vi "CSV_Reader_v1.vi"(8 "error in (no error)":errorcluster, 11 "CSV Reader Inputs":T2={"Frequency Type"=enum."Frequency", "Measurement Type"=enum."Power", "Digital Channel Selector"=enum."2", "Format Type"=enum."Format B", "CSV File Input"=path ""}) -> (0 "error out":errorcluster, 3 "Terminals":T1[](array[typedef]))   [LabVIEW 2017]
uses:
  CSV Reader Inputs.ctl
  Frequency_Type.ctl
  Measurement_Type.ctl
  Digital Channel Selector.ctl
  Terminal Data v1.ctl
  <vilib>/Utility/file.llb/Read Delimited Spreadsheet (string).vi
panel:
  in  "stop":bool
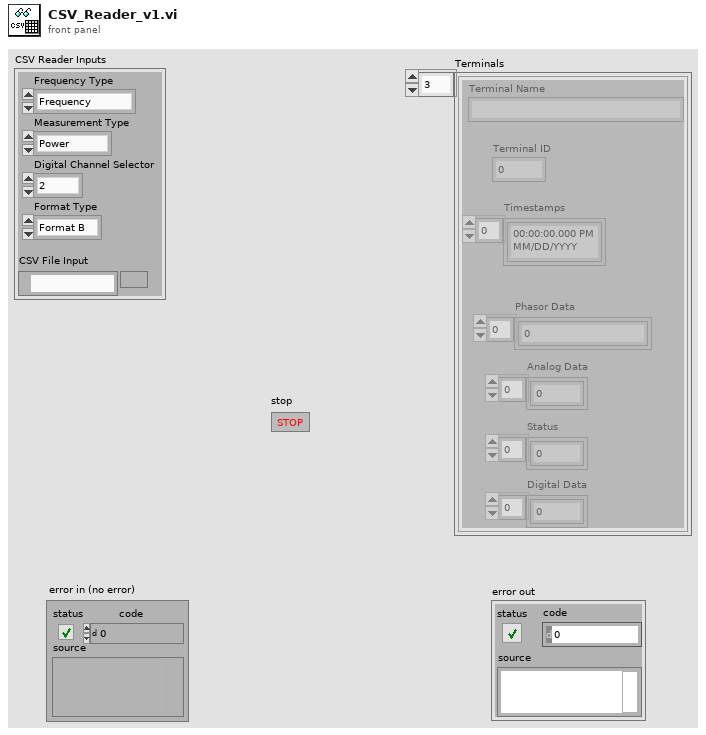
[diagram p1: front panel]
types:
  T1 = typedef "Terminal Data v1.ctl" = cluster{"Terminal Name":string, "Terminal ID":dbl, "Timestamps":timestamp[], "Phasor Data":cdb[], "Analog Data":dbl[], "Status":dbl[], "Digital Data":dbl[]}
  T2 = typedef "CSV Reader Inputs.ctl" = cluster{"Frequency Type":T3, "Measurement Type":T4, "Digital Channel Selector":T5, "Format Type":enum16{"Format A", "Format B"}, "CSV File Input":path}
  T3 = typedef "Frequency_Type.ctl" = enum16{"Frequency", "df/dt"}
  T4 = typedef "Measurement_Type.ctl" = enum16{"Voltage", "Current", "Power"}
  T5 = typedef "Digital Channel Selector.ctl" = enum16{"1", "2", "3"}
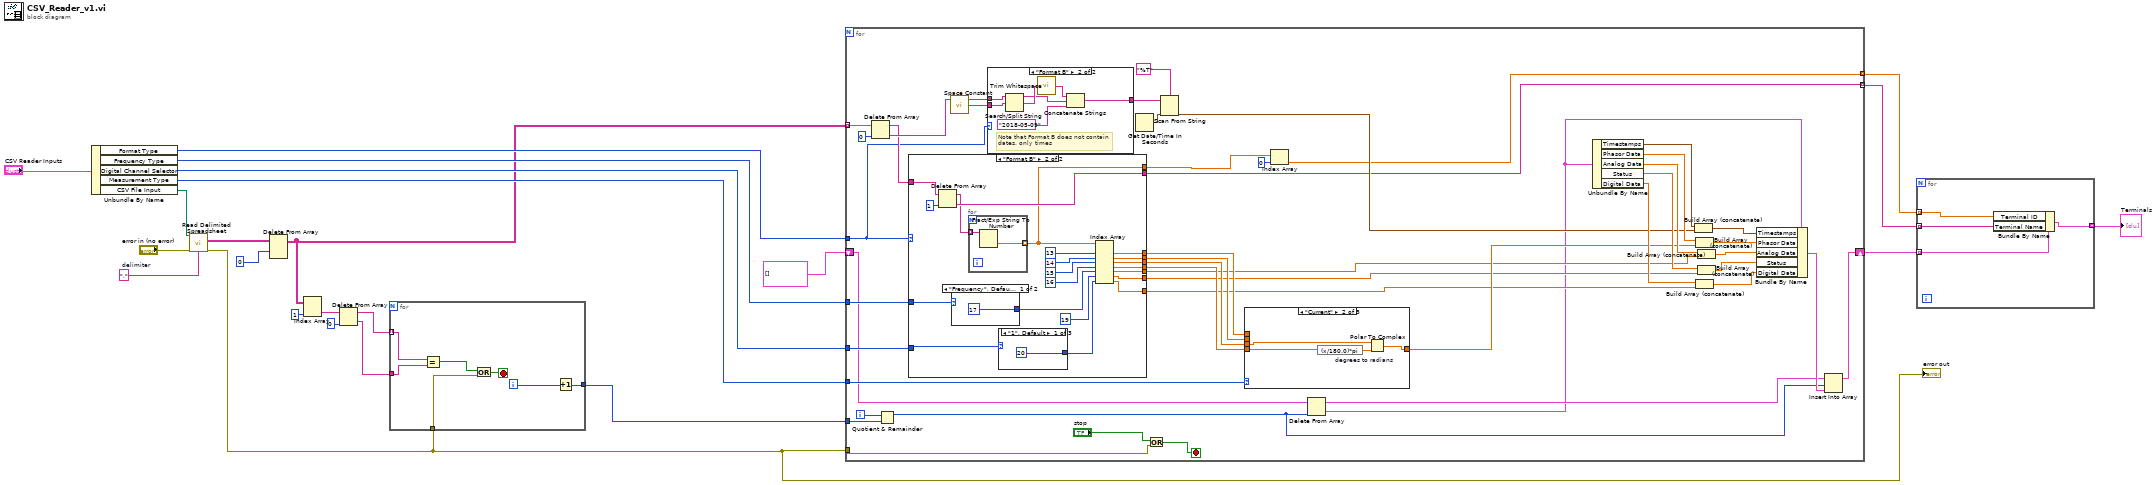
[diagram p0: block diagram]
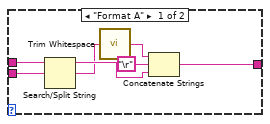
[diagram p2: hidden frame]
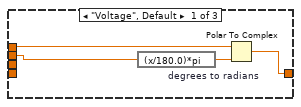
[diagram p3: hidden frame]
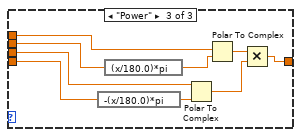
[diagram p4: hidden frame]
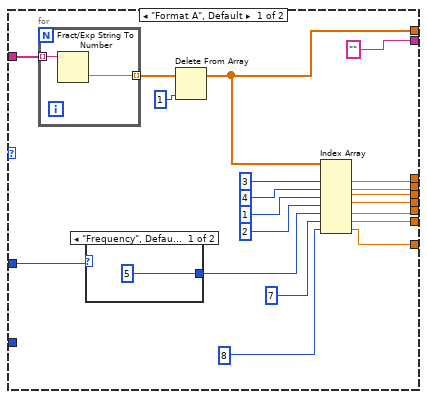
[diagram p5: hidden frame]
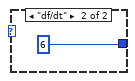
[diagram p6: hidden frame]
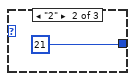
[diagram p7: hidden frame]
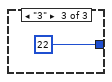
[diagram p8: hidden frame]
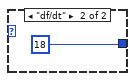
[diagram p9: hidden frame]
diagram:
  w23 = ","  # delimiter
  n1 = Unbundle By Name("CSV Reader Inputs") -> ("Format Type"=w19:enum16{"Format A", "Format B"}, "Frequency Type"=w18:T3, "Digital Channel Selector"=w17:T5, "Measurement Type"=w16:T4, "CSV File Input"=w1:path)
  n2 = call-poly <vilib>:"Read Delimited Spreadsheet.vi"("file path (dialog if empty)"=w1, "error in (no error)"="error in (no error)", "delimiter (\\t)"=w23) -> ("all rows"=w22:string[][], "error out"=w7:errorcluster)  [unwired: 7 in, 4 out]
  "error out" <- w7
  n3 = Delete From Array(array=w22, index (row)=0) -> (array with subset deleted=w14:string[][])  [unwired: 2 in, 1 out]
  n4 = Index Array(array=w14, index (col)=1 ("disabled index (col)")) -> (element=w12:string[])  [unwired: 1 in]
  n5 = Delete From Array(array=w12, index=0) -> (deleted portion=w9:string, array with subset deleted=w10:string[])  [unwired: 1 in]
  n6 = for {
    tunnel: w10 -> [w28] mode=indexing
    tunnel: w9 -> [w27]
    tunnel: [w29] -> w8
    tunnel: w7 -> [w26]
    i -> [w30]
    stop <- w24 stop-if-true
    n7 = Equal?(x=w28, y=w27) -> (x = y?=w25:bool)
    n8 = Or(x=w25, y=w26) -> (x .or. y?=w24:bool)
    n9 = Increment(x=w30) -> (x+1=w29:i32)
  }
  n10 = for {
    tunnel: w14 -> [w72] mode=indexing
    tunnel: w19 -> [w31]
    tunnel: w16 -> [w66]
    tunnel: w18 -> [w61]
    tunnel: w17 -> [w60]
    tunnel: w7 -> [w37]
    shift-right: [w43] -> w5
    shift-left: T1[] [] ("Terminals 2") -> [w41]
    tunnel: w8 -> [w39]
    tunnel: [w33] -> w3 mode=indexing
    tunnel: [w32] -> w4 mode=indexing
    i -> [w45]
    stop <- w36 stop-if-true
    n11 = Delete From Array(array=w72, index=0) -> (deleted portion=w70:string, array with subset deleted=w69:string[])  [unwired: 1 in]
    n12 = Quotient & Remainder(x=w45, y=w39) -> (x-y*floor(x/y)=w40:i32)  [unwired: 1 out]
    n13 = case shown="\"Format B\"" w31 {
      tunnel: w69 -> [w127 w151]
      tunnel: ["" ("String") w150] -> w32
      tunnel: [w108 w148] -> w68
      tunnel: [w118 w143] -> w65
      tunnel: [w117 w142] -> w64
      tunnel: [w116 w141] -> w63
      tunnel: [w115 w140] -> w62
      tunnel: w61 -> [w119 w139]
      tunnel: [w114 w137] -> w51
      tunnel: w60 -> [_ w135]
      tunnel: [w113 w133] -> w49
      tunnel: [w112 w132] -> w47
      frame "Format A", Default {
        n14 = for {
          tunnel: [w130] -> w110 mode=indexing
          tunnel: w127 -> [w131] mode=indexing
          n15 = Fract/Exp String To Number(string=w131) -> (number=w130:dbl)  [unwired: 3 in, 1 out]
        }
        n16 = case shown="\"Frequency\", Default" w119 {
          tunnel: [5 ("index") 6 ("index")] -> w121
          frame "Frequency", Default {
          }
          frame "df/dt" {
          }
        }
        n17 = Delete From Array(array=w110, index=1) -> (array with subset deleted=w108:dbl[])  [unwired: 1 in, 1 out]
        n18 = Index Array(array=w108, index #1=3 ("index"), index #2=4 ("index"), index #3=1 ("index"), index #4=2 ("index"), index #5=w121, index #6=7 ("index"), index #7=8 ("index")) -> (element #1=w118:dbl, element #2=w117:dbl, element #3=w116:dbl, element #4=w115:dbl, element #5=w114:dbl, element #6=w113:dbl, element #7=w112:dbl)
      }
      frame "Format B" {
        n19 = Delete From Array(array=w151, index=1) -> (deleted portion=w150:string, array with subset deleted=w149:string[])  [unwired: 1 in]
        n20 = case shown="\"Frequency\", Default" w139 {
          tunnel: [17 ("index") 18 ("index")] -> w138
          frame "Frequency", Default {
          }
          frame "df/dt" {
          }
        }
        n21 = for {
          tunnel: [w158] -> w148 mode=indexing
          tunnel: w149 -> [w159] mode=indexing
          n22 = Fract/Exp String To Number(string=w159) -> (number=w158:dbl)  [unwired: 3 in, 1 out]
        }
        n23 = case shown="\"1\", Default" w135 {
          tunnel: [20 ("index") 21 ("index") 22 ("index")] -> w134
          frame "1", Default {
          }
          frame "2" {
          }
          frame "3" {
          }
        }
        n24 = Index Array(array=w148, index #1=13 ("index"), index #2=14 ("index"), index #3=15 ("index"), index #4=16 ("index"), index #5=w138, index #6=19 ("index"), index #7=w134) -> (element #1=w143:dbl, element #2=w142:dbl, element #3=w141:dbl, element #4=w140:dbl, element #5=w137:dbl, element #6=w133:dbl, element #7=w132:dbl)
      }
    }
    n25 = call <vilib>:"Space Constant.vi"() -> ("String"=w75:string)
    n26 = case shown="\"Format B\"" w31 {
      tunnel: [w83 w85] -> w76
      tunnel: w75 -> [w79 w88]
      tunnel: w70 -> [w77 w87]
      frame "Format A" {
        n27 = Search/Split String(string=w77, search string/char (-)=w79) -> (substring before match=w81:string, match + rest of string=w80:string)  [unwired: 1 in, 1 out]
        n28 = call <vilib>:"Trim Whitespace.vi"("string"=w80) -> ("trimmed string"=w82:string)  [unwired: 1 in]
        n29 = Concatenate Strings(w82, "\r", w81) -> (w83:string)
      }
      frame "Format B" {
        # "Note that Format B does not contain \ndates, only times"
        n30 = Search/Split String(string=w87, search string/char (-)=w88) -> (substring before match=w86:string, match + rest of string=w89:string)  [unwired: 1 in, 1 out]
        n31 = call <vilib>:"Trim Whitespace.vi"("string"=w89) -> ("trimmed string"=w90:string)  [unwired: 1 in]
        n32 = Concatenate Strings(w90, w86, "2018-05-09" ("string")) -> (w85:string)
      }
    }
    n33 = Get Date/Time In Seconds() -> (seconds since 1Jan1904=w74:timestamp)
    n34 = Or(x="stop", y=w37) -> (x .or. y?=w36:bool)
    n35 = Scan From String(format string="%T", input string=w76, default 1=w74) -> (output 1=w54:timestamp)  [unwired: 2 in, 3 out]
    n36 = case shown="\"Current\"" w66 {
      tunnel: w65 -> [w93 _ w103]
      tunnel: w64 -> [w92 _ w102]
      tunnel: w63 -> [_ w96 w101]
      tunnel: w62 -> [_ w95 w100]
      tunnel: [w91 w97 w99] -> w53
      frame "Voltage", Default {
        n37 = expression code="(x/180.0)*pi" "degrees to radians"(w92) -> (w94:dbl)
        n38 = Polar To Complex(1:w94, 2:w93) -> (0:w91:cdb)
      }
      frame "Current" {
        n39 = expression code="(x/180.0)*pi" "degrees to radians"(w95) -> (w98:dbl)
        n40 = Polar To Complex(1:w98, 2:w96) -> (0:w97:cdb)
      }
      frame "Power" {
        n41 = expression code="-(x/180.0)*pi" ("degrees to radians")(w100) -> (w107:dbl)
        n42 = expression code="(x/180.0)*pi" ("degrees to radians")(w102) -> (w105:dbl)
        n43 = Polar To Complex(1:w107, 2:w101) -> (0:w106:cdb)
        n44 = Polar To Complex(1:w105, 2:w103) -> (0:w104:cdb)
        n45 = Multiply(x=w104, y=w106) -> (x*y=w99:cdb)
      }
    }
    n46 = Index Array "Index Array"(array=w68, index=0) -> (element=w33:dbl)
    n47 = Delete From Array(array=w41, index=w40) -> (deleted portion=w34:T1, array with subset deleted=w38:T1[])  [unwired: 1 in]
    n48 = Unbundle By Name(w34) -> ("Timestamps"=w59:timestamp[], "Phasor Data"=w58:cdb[], "Analog Data"=w57:dbl[], "Status"=w56:dbl[], "Digital Data"=w55:dbl[])
    n49 = Build Array (concatenate)(w59, w54) -> (w44:timestamp[])
    n50 = Build Array (concatenate)(w58, w53) -> (w52:cdb[])
    n51 = Build Array (concatenate)(w55, w47) -> (w46:dbl[])
    n52 = Build Array (concatenate)(w56, w49) -> (w48:dbl[])
    n53 = Build Array (concatenate)(w57, w51) -> (w50:dbl[])
    n54 = Bundle By Name(cluster=w34, "Timestamps"=w44, "Phasor Data"=w52, "Analog Data"=w50, "Status"=w48, "Digital Data"=w46) -> (w42:T1)
    n55 = Insert Into Array(array=w38, index=w40, new element=w42) -> (w43:T1[])
  }
  n56 = for {
    tunnel: w5 -> [w161] mode=indexing
    tunnel: w4 -> [w162] mode=indexing
    tunnel: w3 -> [w163] mode=indexing
    tunnel: [w160] -> w2 mode=indexing
    n57 = Bundle By Name(cluster=w161, "Terminal ID"=w163, "Terminal Name"=w162) -> (w160:T1)
  }
  "Terminals" <- w2
